vi "simulacao_robo_movel.vi"() -> ()   [LabVIEW 2013]
panel:
  out "Tank":dbl(slide) scale=0.0..1000.0
  out "Entrada":dbl(knob) scale=0.0..1000.0
  out "Vo":dbl(graph)
  in  "Vi":dbl(knob) scale=0.0..10.0
  in  "stop":bool
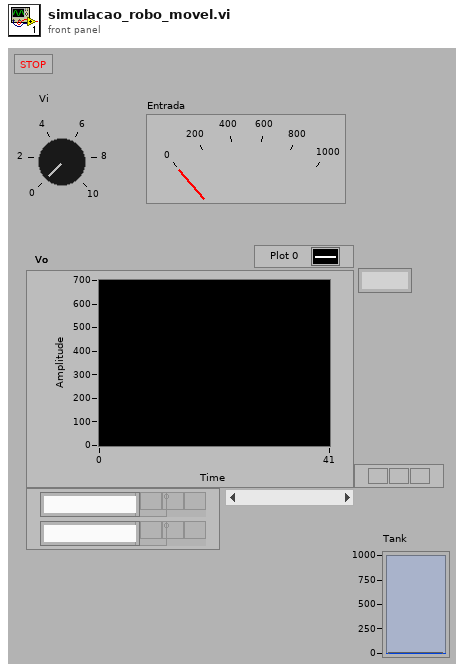
[diagram p1: front panel]
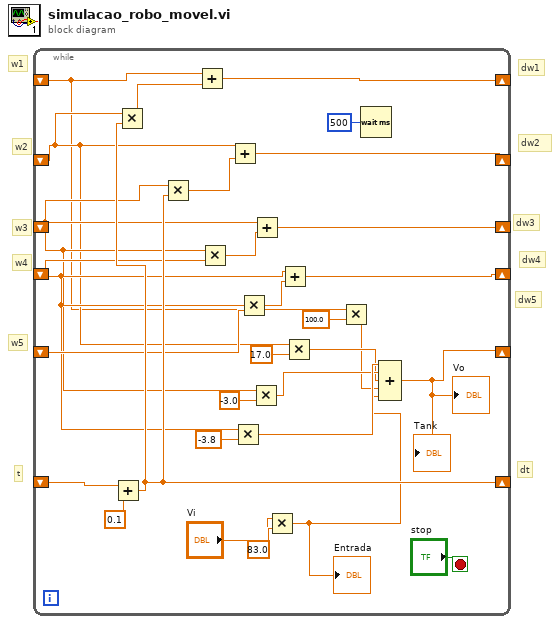
[diagram p0: block diagram]
diagram:
  # "t"
  # "dt"
  # "dw5"
  # "dw4"
  # "dw3"
  # "dw2"
  # "dw1"
  # "w1"
  # "w5"
  # "w4"
  # "w3"
  # "w2"
  n1 = while {
    shift-right: [w25] -> _
    shift-left: _ -> [w28]
    shift-right: [w27] -> _
    shift-left: _ -> [w6]
    shift-right: [w24] -> _
    shift-left: _ -> [w10]
    shift-right: [w22] -> _
    shift-left: _ -> [w13]
    shift-right: [w20] -> _
    shift-left: _ -> [w16]
    shift-right: [w1] -> _
    shift-left: _ -> [w19]
    stop <- "stop" stop-if-true
    n2 = Add(x=w28, y=0.1) -> (x+y=w25:dbl)
    n3 = Multiply(x=w10, y=w25) -> (x*y=w26:dbl)
    n4 = Multiply(x=w13, y=w25) -> (x*y=w23:dbl)
    n5 = Add(x=w6, y=w26) -> (x+y=w27:dbl)
    n6 = Multiply(x=w13, y=w16) -> (x*y=w21:dbl)
    n7 = Add(x=w10, y=w23) -> (x+y=w24:dbl)
    n8 = Multiply(x=w16, y=-3.8) -> (x*y=w15:dbl)
    n9 = Multiply(x=w16, y=w19) -> (x*y=w18:dbl)
    n10 = Multiply(x=w13, y=-3.0) -> (x*y=w12:dbl)
    n11 = Add(x=w13, y=w21) -> (x+y=w22:dbl)
    n12 = Multiply(x="Vi", y=83.0) -> (x*y=w2:dbl)
    "Entrada" <- w2
    n13 = Add(x=w16, y=w18) -> (x+y=w20:dbl)
    n14 = Multiply(x=w10, y=17.0) -> (x*y=w9:dbl)
    n15 = Multiply(x=w6, y=100.0) -> (x*y=w7:dbl)
    n16 = Wait (ms)(milliseconds to wait=u32 500) -> ()  [unwired: 1 out]
    n17 = Compound Arithmetic op=ADD(w15, w12, w9, w7, w2) -> (w1:dbl)
    "Vo" <- w1
    "Tank" <- w1
  }
